vi "TESTER_v1.vi"() -> ()   [LabVIEW 2014, in "PICam.lvlib"]
uses:
  PICam.lvlib
  Ctrls/PicamModel.ctl
  Ctrls/PicamROI.ctl
  Ctrls/ShutterTimingMode.ctl
  Ctrls/PicamAdcQuality.ctl
  Ctrls/PicamADCAnalogGain.ctl
  Ctrls/PicamTriggerResponse.ctl
  Ctrls/PicamTriggerDetermination.ctl
  Ctrls/PicamOutputSignal.ctl
  Ctrls/PicamPixelFormat.ctl
  Ctrls/ReadoutControlMode.ctl
  Ctrls/PicamReadoutOrientation.ctl
  Ctrls/PicamSensorType.ctl
  Ctrls/PicamTimeStamps.ctl
  Ctrls/PicamSensorTemperatureStatus.ctl
  Ctrls/PicamCcdCharacteristics.ctl
  Ctrls/PicamOrientation.ctl
panel:
  in  "PicamTriggerDetemination":T1=2 items=["PositivePolarity"=1, "NegativePolarity"=2, "RisingEdge"=3, "FallingEdge"=4, "AlternatingEdgeRising"=5, "AlternatingEdgeFalling"=6]
  in  "PicamTriggerResponse":T2=1 items=["NoResponse"=1, "ReadoutPerTrigger"=2, "ShiftPerTrigger"=3, "ExposeDuringTriggerPulse"=4, "StartOnSingleTrigger"=5, "GatePerTrigger"=6]
  in  "PicamOutputSignal_":T3=2 items=["NotReadingOut"=1, "ShutterOpen"=2, "Busy"=3, "AlwaysLow"=4, "AlwaysHigh"=5, "Acquiring"=6, "ShiftingUnderMask"=7, "Exposing"=8, "EffectivelyExposing"=9, "ReadingOut"=10, "WaitingForTrigger"=11, "InternalTriggerT0"=12, "Gate"=13, "AuxOutput"=14, "EffectivelyExposingAlternation"=15]
  in  "ReadoutControlMode":T4=1 items=["FullFrame"=1, "FrameTransfer"=2, "Kinetics"=3, "SpectraKinetics"=4, "Interline"=5, "Dif"=6, "SeNsR"=7, "RollingShutter"=8]
  in  "PicamTimeStamps_":T5 items=["None", "ExposureStarted", "ExposureEnded"]
  in  "PicamAdcAnalogGain":T6=2 items=["Low"=1, "Medium"=2, "High"=3]
  in  "PicamAdcQuality":T7=1 items=["LowNoise"=1, "HighCapacity"=2, "ElectronMultiplied"=3, "HighSpeed"=4]
  in  "ShutterTimingMode":T8=1 items=["Normal"=1, "AlwaysClosed"=2, "AlwaysOpen"=3, "OpenBeforeTrigger"=4]
  in  "ReadoutCount":i64=1
  in  "TimeStampResolution":i32=10000000
  in  "CleanUntilTrigger":bool=TRUE
  in  "CleanSerialRegister":bool=TRUE
  in  "TrackFrames":bool
  in  "DisableDataFormatting":bool
  in  "NormalizeOrientation":bool=TRUE
  in  "CleanSectionFinalHeightCount":i32=5
  in  "CleanSectionFinalHeight":i32=2
  in  "CleanCycleHeight":i32=100
  in  "CleanCycleCount":i32=1
  in  "ActiveBottomMargin":i32
  in  "ActiveRightMargin":i32=8
  in  "ActiveTopMargin":i32
  in  "ActiveLeftMargin":i32=8
  in  "ActiveHeight":i32=100
  in  "ActiveWidth":i32=1340
  in  "FrameTrackingBitDepth":i32=64
  in  "TimeStampBitDepth":i32=64
  in  "AdcBitDepth":i32=2
  in  "KineticsWindowHeight":i32=10
  in  "VerticalShiftRate":dbl=15.2
  in  "ShutterClosingDelay":dbl=8.0
  in  "ShutterDelayResolution":dbl=1000.0
  in  "AdcSpeed":dbl=2.0
  in  "SensorTemperatureSetPoint (C)":dbl=-75.0
  in  "ExposureTime (ms)":dbl=300.0
  in  "SET PARAMETERS?":bool
  out "rois":T9[](array[typedef])=[{"x"=1, "width"=1339, "x_binning"=1, "y"=1, "height"=99, "y_binning"=1}]
  out "ExactReadoutCountMaximum":i64=65534
  out "TimeStampResolution":i64=10000000
  out "ReadoutCount":i64=1
  out "TrackFrames":bool
  out "NormalizeOrientation":bool=TRUE
  out "CleanUntilTrigger":bool=TRUE
  out "CleanSerialRegister":bool=TRUE
  out "DisableDataFormatting":bool
  out "Orientation":T10 items=["Normal", "FlippedHorizontally", "FlippedVertically"]
  out "PicamCcdCharacteristics_":T11=3 items=["None", "BackIlluminated", "DeepDepleted", "OpenElectrode", "UVEnhanced", "ExcelonEnabled", "SecondaryMask", "Multiport", "AdvancedInvertedMode", "HighResistivity"]
  out "SensorTemperatureStatus":T12=2 items=["Unlocked"=1, "Locked"=2, "Faulted"=3]
  out "TimeStamps":T5 items=["None", "ExposureStarted", "ExposureEnded"]
  out "Sensor Type":T13=1 items=["CCD"=1, "InGaAs"=2, "CMOS"=3]
  out "ReadoutOrientation_":T14 items=["Normal", "FlippedHorizontally", "FlippedVertically"]
  out "ReadoutControlMode":T4=1 items=["FullFrame"=1, "FrameTransfer"=2, "Kinetics"=3, "SpectraKinetics"=4, "Interline"=5, "Dif"=6, "SeNsR"=7, "RollingShutter"=8]
  out "Pixel Format":T15=1 items=["Monochrome16Bit"=1, "Monochrome32Bit"=2]
  out "SensorTemperatureReading":dbl=-75.0
  out "ReadoutTimeCalculation":dbl=69.37595
  out "ReadoutRateCalculation":dbl=12.923912404306506
  out "PixelWidth":dbl=20.0
  out "PixelHeight":dbl=20.0
  out "PixelGapWidth":dbl
  out "PixelGapHeight":dbl
  out "SensorTemperatureSetPoint":dbl=-75.0
  out "VerticalShiftRate":dbl=15.2
  out "FrameRateCalculation":dbl=12.923912404306506
  out "OnlineReadoutRateCalculation":dbl=12.923912404306506
  out "SensorSecondaryMaskedHeight":i32
  out "SensorSecondaryActiveHeight":i32
  out "SensorMaskedTopMargin":i32
  out "SensorMaskedHeight":i32
  out "SensorMaskedBottomMargin":i32
  out "SensorActiveTopMargin":i32
  out "SensorActiveRightMargin":i32=8
  out "SensorActiveLeftMargin":i32=8
  out "SensorActiveExtendedHeight":i32
  out "SensorActiveBottomMargin":i32
  out "ReadoutStride":i32=265122
  out "PixelBitDepth":i32=16
  out "KineticsWindowHeight":i32=10
  out "FrameTrackingBitDepth":i32=64
  out "FrameStride":i32=265122
  out "FramesPerReadout":i32=1
  out "FrameSize":i32=265122
  out "CleanSectionFinalHeightCount":i32=5
  out "CleanSectionFinalHeight":i32=2
  out "Active Width":i32=1340
  out "ActiveTopMargin":i32
  out "ActiveRightMargin":i32=8
  out "ActiveLeftMargin":i32=8
  out "Active Height":i32=100
  out "CleanCycleCount":i32=1
  out "CleanCycleHeight":i32=100
  out "ActiveBottomMargin":i32
  out "TimestampBitDepth":i32=64
  out "OutputSignal":T3=2 items=["NotReadingOut"=1, "ShutterOpen"=2, "Busy"=3, "AlwaysLow"=4, "AlwaysHigh"=5, "Acquiring"=6, "ShiftingUnderMask"=7, "Exposing"=8, "EffectivelyExposing"=9, "ReadingOut"=10, "WaitingForTrigger"=11, "InternalTriggerT0"=12, "Gate"=13, "AuxOutput"=14, "EffectivelyExposingAlternation"=15]
  out "PicamTriggerDetemination_":T1=2 items=["PositivePolarity"=1, "NegativePolarity"=2, "RisingEdge"=3, "FallingEdge"=4, "AlternatingEdgeRising"=5, "AlternatingEdgeFalling"=6]
  out "PicamTriggerResponse_":T2=1 items=["NoResponse"=1, "ReadoutPerTrigger"=2, "ShiftPerTrigger"=3, "ExposeDuringTriggerPulse"=4, "StartOnSingleTrigger"=5, "GatePerTrigger"=6]
  out "AdcBitDepth":i32
  out "AdcSpeed":dbl=2.0
  out "Sensor Active Width":i32=1340
  out "PicamAdcAnalogGain":T6=2 items=["Low"=1, "Medium"=2, "High"=3]
  out "PicamAdcQuality":T7=1 items=["LowNoise"=1, "HighCapacity"=2, "ElectronMultiplied"=3, "HighSpeed"=4]
  out "Shutter Delay Resolution":dbl=1000.0
  out "Shutter Closing Delay":dbl=8.0
  out "Shutter Timing Mode":T8=1 items=["Normal"=1, "AlwaysClosed"=2, "AlwaysOpen"=3, "OpenBeforeTrigger"=4]
  out "Sensor Active Height":i32=100
  out "Exposure Time":dbl
  out "Raw CCD data":u16[][](graph)
  out "Total pixel number":i32=132561
  in  "PicamROI":T9={"x"=1, "width"=1339, "x_binning"=1, "y"=1, "height"=99, "y_binning"=1}
  out "Frame size (bytes)":i32=265122
  out "PicamModel":T16=5 items=["PicamModel_PIMte1024Series"=1401, "PicamModel_PIMte1024F"=1402, "PicamModel_PIMte1024B"=1403, "PicamModel_PIMte1024BR"=1405, "PicamModel_PIMte1024BUV"=1404, "PicamModel_PIMte1024FTSeries"=1406, "PicamModel_PIMte1024FT"=1407, "PicamModel_PIMte1024BFT"=1408, "PicamModel_PIMte1300Series"=1412, "PicamModel_PIMte1300B"=1413, "PicamModel_PIMte1300R"=1414, "PicamModel_PIMte1300BR"=1415, "PicamModel_PIMte2048Series"=1416, "PicamModel_PIMte2048B"=1417, "PicamModel_PIMte2048BR"=1418, "PicamModel_PIMte2KSeries"=1409, "PicamModel_PIMte2KB"=1410, "PicamModel_PIMte2KBUV"=1411, "PicamModel_PixisSeries"=0, "PicamModel_Pixis100Series"=1, "PicamModel_Pixis100F"=2, "PicamModel_Pixis100B"=6, "PicamModel_Pixis100R"=3, "PicamModel_Pixis100C"=4, "PicamModel_Pixis100BR"=5, "PicamModel_Pixis100BExcelon"=54, "PicamModel_Pixis100BRExcelon"=55, "PicamModel_PixisXO100B"=7, "PicamModel_PixisXO100BR"=8, "PicamModel_PixisXB100B"=68, "PicamModel_PixisXB100BR"=69, "PicamModel_Pixis256Series"=26, "PicamModel_Pixis256F"=27, "PicamModel_Pixis256B"=29, "PicamModel_Pixis256E"=28, "PicamModel_Pixis256BR"=30, "PicamModel_PixisXB256BR"=31, "PicamModel_Pixis400Series"=37, "PicamModel_Pixis400F"=38, "PicamModel_Pixis400B"=40, "PicamModel_Pixis400R"=39, "PicamModel_Pixis400BR"=41, "PicamModel_Pixis400BExcelon"=56, "PicamModel_Pixis400BRExcelon"=57, "PicamModel_PixisXO400B"=42, "PicamModel_PixisXB400BR"=70, "PicamModel_Pixis512Series"=43, "PicamModel_Pixis512F"=44, "PicamModel_Pixis512B"=45, "PicamModel_Pixis512BUV"=46, "PicamModel_Pixis512BExcelon"=58, "PicamModel_PixisXO512F"=49, "PicamModel_PixisXO512B"=50, "PicamModel_PixisXF512F"=48, "PicamModel_PixisXF512B"=47, "PicamModel_Pixis1024Series"=9, "PicamModel_Pixis1024F"=10, "PicamModel_Pixis1024B"=11, "PicamModel_Pixis1024BR"=13, "PicamModel_Pixis1024BUV"=12, "PicamModel_Pixis1024BExcelon"=59, "PicamModel_Pixis1024BRExcelon"=60, "PicamModel_PixisXO1024F"=16, "PicamModel_PixisXO1024B"=14, "PicamModel_PixisXO1024BR"=15, "PicamModel_PixisXF1024F"=17, "PicamModel_PixisXF1024B"=18, "PicamModel_PixisXB1024BR"=71, "PicamModel_Pixis1300Series"=51, "PicamModel_Pixis1300F"=52, "PicamModel_Pixis1300F_2"=75, "PicamModel_Pixis1300B"=53, "PicamModel_Pixis1300BR"=73, "PicamModel_Pixis1300BExcelon"=61, "PicamModel_Pixis1300BRExcelon"=62, "PicamModel_PixisXO1300B"=65, "PicamModel_PixisXF1300B"=66, "PicamModel_PixisXB1300R"=72, "PicamModel_Pixis2048Series"=20, "PicamModel_Pixis2048F"=21, "PicamModel_Pixis2048B"=22, "PicamModel_Pixis2048BR"=67, "PicamModel_Pixis2048BExcelon"=63, "PicamModel_Pixis2048BRExcelon"=74, "PicamModel_PixisXO2048B"=23, "PicamModel_PixisXF2048F"=25, "PicamModel_PixisXF2048B"=24, "PicamModel_Pixis2KSeries"=32, "PicamModel_Pixis2KF"=33, "PicamModel_Pixis2KB"=34, "PicamModel_Pixis2KBUV"=36, "PicamModel_Pixis2KBExcelon"=64, "PicamModel_PixisXO2KB"=35, "PicamModel_QuadroSeries"=100, "PicamModel_Quadro4096"=101, "PicamModel_Quadro4096_2"=103, "PicamModel_Quadro4320"=102, "PicamModel_ProEMSeries"=200, "PicamModel_ProEM512Series"=203, "PicamModel_ProEM512B"=201, "PicamModel_ProEM512BK"=205, "PicamModel_ProEM512BExcelon"=204, "PicamModel_ProEM512BKExcelon"=206, "PicamModel_ProEM1024Series"=207, "PicamModel_ProEM1024B"=202, "PicamModel_ProEM1024BExcelon"=208, "PicamModel_ProEM1600Series"=209, "PicamModel_ProEM1600xx2B"=212, "PicamModel_ProEM1600xx2BExcelon"=210, "PicamModel_ProEM1600xx4B"=213, "PicamModel_ProEM1600xx4BExcelon"=211, "PicamModel_ProEMPlusSeries"=600, "PicamModel_ProEMPlus512Series"=603, "PicamModel_ProEMPlus512B"=601, "PicamModel_ProEMPlus512BK"=605, "PicamModel_ProEMPlus512BExcelon"=604, "PicamModel_ProEMPlus512BKExcelon"=606, "PicamModel_ProEMPlus1024Series"=607, "PicamModel_ProEMPlus1024B"=602, "PicamModel_ProEMPlus1024BExcelon"=608, "PicamModel_ProEMPlus1600Series"=609, "PicamModel_ProEMPlus1600xx2B"=612, "PicamModel_ProEMPlus1600xx2BExcelon"=610, "PicamModel_ProEMPlus1600xx4B"=613, "PicamModel_ProEMPlus1600xx4BExcelon"=611, "PicamModel_ProEMHSSeries"=1200, "PicamModel_ProEMHS512Series"=1201, "PicamModel_ProEMHS512B"=1202, "PicamModel_ProEMHS512BK"=1207, "PicamModel_ProEMHS512BExcelon"=1203, "PicamModel_ProEMHS512BKExcelon"=1208, "PicamModel_ProEMHS1024Series"=1204, "PicamModel_ProEMHS1024B"=1205, "PicamModel_ProEMHS1024BExcelon"=1206, "PicamModel_ProEMHS1024B_2"=1212, "PicamModel_ProEMHS1024BExcelon_2"=1213, "PicamModel_ProEMHS1024B_3"=1214, "PicamModel_ProEMHS1024BExcelon_3"=1215, "PicamModel_ProEMHS1K10Series"=1209, "PicamModel_ProEMHS1KB10"=1210, "PicamModel_ProEMHS1KB10Excelon"=1211, "PicamModel_PIMax3Series"=300, "PicamModel_PIMax31024I"=301, "PicamModel_PIMax31024x256"=302, "PicamModel_PIMax4Series"=700, "PicamModel_PIMax41024ISeries"=703, "PicamModel_PIMax41024I"=701, "PicamModel_PIMax41024IRF"=704, "PicamModel_PIMax41024FSeries"=710, "PicamModel_PIMax41024F"=711, "PicamModel_PIMax41024FRF"=712, "PicamModel_PIMax41024x256Series"=705, "PicamModel_PIMax41024x256"=702, "PicamModel_PIMax41024x256RF"=706, "PicamModel_PIMax42048Series"=716, "PicamModel_PIMax42048F"=717, "PicamModel_PIMax42048B"=718, "PicamModel_PIMax42048FRF"=719, "PicamModel_PIMax42048BRF"=720, "PicamModel_PIMax4512EMSeries"=708, "PicamModel_PIMax4512EM"=707, "PicamModel_PIMax4512BEM"=709, "PicamModel_PIMax41024EMSeries"=713, "PicamModel_PIMax41024EM"=715, "PicamModel_PIMax41024BEM"=714, "PicamModel_PylonSeries"=400, "PicamModel_Pylon100Series"=418, "PicamModel_Pylon100F"=404, "PicamModel_Pylon100B"=401, "PicamModel_Pylon100BR"=407, "PicamModel_Pylon100BExcelon"=425, "PicamModel_Pylon100BRExcelon"=426, "PicamModel_Pylon256Series"=419, "PicamModel_Pylon256F"=409, "PicamModel_Pylon256B"=410, "PicamModel_Pylon256E"=411, "PicamModel_Pylon256BR"=412, "PicamModel_Pylon400Series"=420, "PicamModel_Pylon400F"=405, "PicamModel_Pylon400B"=402, "PicamModel_Pylon400BR"=408, "PicamModel_Pylon400BExcelon"=427, "PicamModel_Pylon400BRExcelon"=428, "PicamModel_Pylon1024Series"=421, "PicamModel_Pylon1024B"=417, "PicamModel_Pylon1024BExcelon"=429, "PicamModel_Pylon1300Series"=422, "PicamModel_Pylon1300F"=406, "PicamModel_Pylon1300B"=403, "PicamModel_Pylon1300R"=438, "PicamModel_Pylon1300BR"=432, "PicamModel_Pylon1300BExcelon"=430, "PicamModel_Pylon1300BRExcelon"=433, "PicamModel_Pylon2048Series"=423, "PicamModel_Pylon2048F"=415, "PicamModel_Pylon2048B"=434, "PicamModel_Pylon2048BR"=416, "PicamModel_Pylon2048BExcelon"=435, "PicamModel_Pylon2048BRExcelon"=436, "PicamModel_Pylon2KSeries"=424, "PicamModel_Pylon2KF"=413, "PicamModel_Pylon2KB"=414, "PicamModel_Pylon2KBUV"=437, "PicamModel_Pylon2KBExcelon"=431, "PicamModel_PylonirSeries"=900, "PicamModel_Pylonir1024Series"=901, "PicamModel_Pylonir102422"=902, "PicamModel_Pylonir102417"=903, "PicamModel_PionirSeries"=500, "PicamModel_Pionir640"=501, "PicamModel_NirvanaSeries"=800, "PicamModel_Nirvana640"=801, "PicamModel_NirvanaSTSeries"=1300, "PicamModel_NirvanaST640"=1301, "PicamModel_NirvanaLNSeries"=1100, "PicamModel_NirvanaLN640"=1101, "PicamModel_SophiaSeries"=1800, "PicamModel_Sophia2048Series"=1801, "PicamModel_Sophia2048B"=1802, "PicamModel_Sophia2048BExcelon"=1803, "PicamModel_SophiaXO2048B"=1804, "PicamModel_SophiaXF2048B"=1805, "PicamModel_SophiaXB2048B"=1806, "PicamModel_Sophia2048135Series"=1807, "PicamModel_Sophia2048135"=1808, "PicamModel_Sophia2048B135"=1809, "PicamModel_Sophia2048BR135"=1810, "PicamModel_Sophia2048B135Excelon"=1811, "PicamModel_Sophia2048BR135Excelon"=1812, "PicamModel_SophiaXO2048B135"=1813, "PicamModel_SophiaXO2048BR135"=1814, "PicamModel_BlazeSeries"=1500, "PicamModel_Blaze100Series"=1507, "PicamModel_Blaze100B"=1501, "PicamModel_Blaze100BR"=1505, "PicamModel_Blaze100HR"=1503, "PicamModel_Blaze100BRLD"=1509, "PicamModel_Blaze100BExcelon"=1511, "PicamModel_Blaze100BRExcelon"=1513, "PicamModel_Blaze100HRExcelon"=1515, "PicamModel_Blaze100BRLDExcelon"=1517, "PicamModel_Blaze400Series"=1508, "PicamModel_Blaze400B"=1502, "PicamModel_Blaze400BR"=1506, "PicamModel_Blaze400HR"=1504, "PicamModel_Blaze400BRLD"=1510, "PicamModel_Blaze400BExcelon"=1512, "PicamModel_Blaze400BRExcelon"=1514, "PicamModel_Blaze400HRExcelon"=1516, "PicamModel_Blaze400BRLDExcelon"=1518, "PicamModel_FergieSeries"=1600, "PicamModel_Fergie256Series"=1601, "PicamModel_Fergie256B"=1602, "PicamModel_Fergie256BR"=1607, "PicamModel_Fergie256BExcelon"=1603, "PicamModel_Fergie256BRExcelon"=1608, "PicamModel_Fergie256FTSeries"=1604, "PicamModel_Fergie256FFT"=1609, "PicamModel_Fergie256BFT"=1605, "PicamModel_Fergie256BRFT"=1610, "PicamModel_Fergie256BFTExcelon"=1606, "PicamModel_Fergie256BRFTExcelon"=1611, "PicamModel_FergieAccessorySeries"=1700, "PicamModel_FergieLampSeries"=1701, "PicamModel_FergieAEL"=1702, "PicamModel_FergieQTH"=1703, "PicamModel_FergieLaserSeries"=1704, "PicamModel_FergieLaser785"=1705, "PicamModel_KuroSeries"=1900, "PicamModel_Kuro1200B"=1901, "PicamModel_Kuro1608B"=1902, "PicamModel_Kuro2048B"=1903]
  out "Camera detected?":bool=TRUE
  out "Serial":string="0205070001"
  out "Sensor name":string="E2V 1340 x 100 (CCD 36)(B)(R)"
  in  "cam index":i32
  out "PICam version":string="5.7.1.1903"
  out "error out":errorcluster
  # "GET INFORMATION / PARAMETER VALUES:"
  # "PIXIS SDK"
  # "Can be set greater than 1340?"
  # "Can be set greater than 100?"
  # "Less important?\n\n- Picam_DestroyString()\n- Picam_GetEnumnerationString()\n- Picam_DestroyCameraIDs()\n- Picam_GetUnavailableCameraIDs()\n+ other Destroy-methods and gettype methods"
  # "To implement:\n\n- Picam_IsLibraryInitialized()\n- Picam_IsCameraIDConnected()\n- Picam_IsCameraIDOpenElsewhere()\n- Picam_DestroyHandles()\n- Picam_GetOpenCameras()\n- Picam_IsCameraConnected()\n- Picam_IsCameraFaulted()\n- Picam_GetFirmwareDetails()\n- Picam_CanSetParameterOnline()\n- Picam_CanReadParameter() \n- Picam_CanWaitForStatusParameter()\n- Picam_GetStatusParameterPurview()\n- Picam_EstimateTimeToStatusParameterValue()\n- Picam_WaitForStatusParameterValue()\n- Picam_CommitParameters()\n- Picam_AreParametersCommited()\n- Picam_WaitForAcquisitionUpdate()\n- PicamAdvanced_GetAcquisitionBuffer()\n- PicamAdvanced_SetAcquisitionBuffer()\n- PicamAdvanced_HasAcquisitionBufferOverrun()"
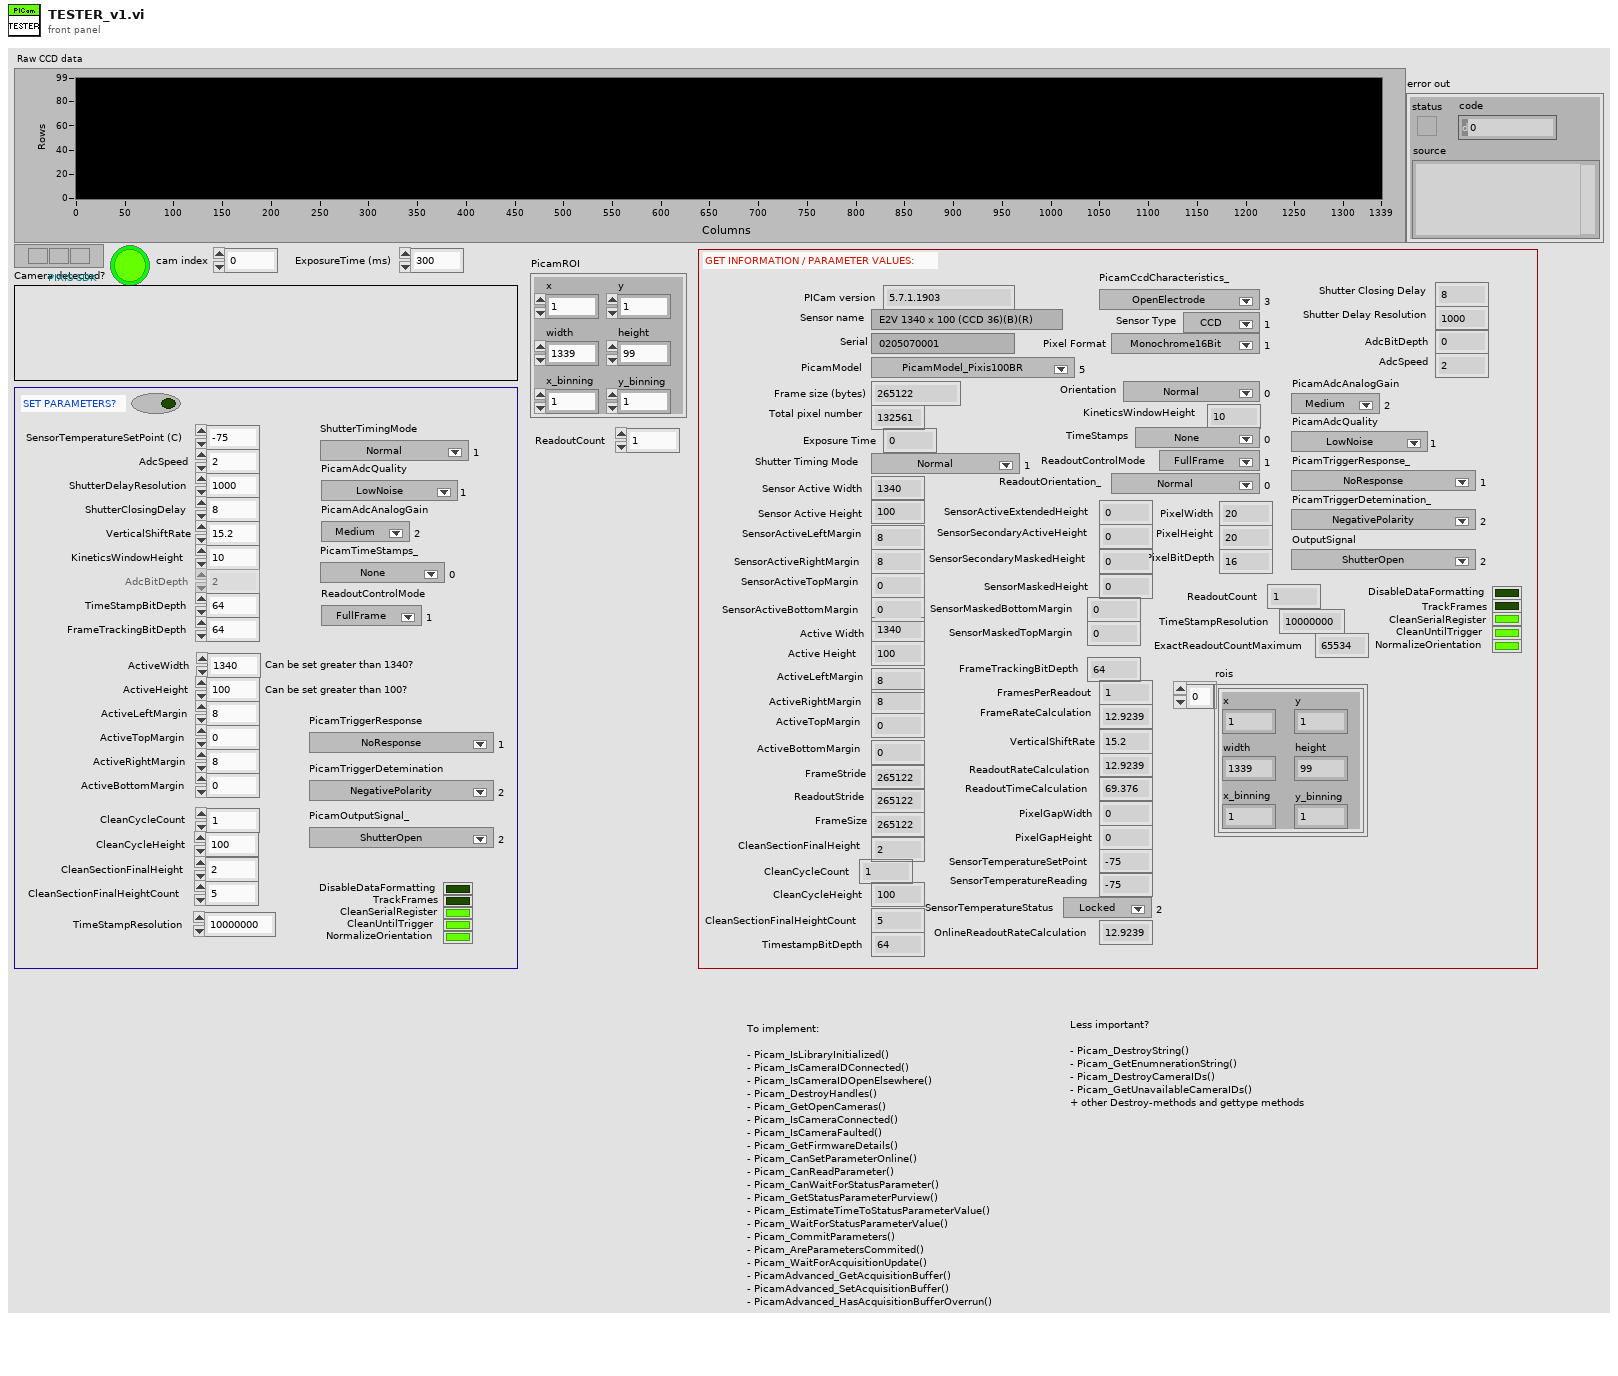
[diagram p1: front panel]
types:
  T1 = typedef "PICam.lvlib/PicamTriggerDetermination.ctl" = u32
  T2 = typedef "PICam.lvlib/PicamTriggerResponse.ctl" = u32
  T3 = typedef "PICam.lvlib/PicamOutputSignal.ctl" = u32
  T4 = typedef "PICam.lvlib/ReadoutControlMode.ctl" = u32
  T5 = typedef "PICam.lvlib/PicamTimeStamps.ctl" = u32
  T6 = typedef "PICam.lvlib/PicamADCAnalogGain.ctl" = u32
  T7 = typedef "PICam.lvlib/PicamAdcQuality.ctl" = u32
  T8 = typedef "PICam.lvlib/ShutterTimingMode.ctl" = u32
  T9 = typedef "PICam.lvlib/PicamROI.ctl" = cluster{"x":i32, "width":i32, "x_binning":i32, "y":i32, "height":i32, "y_binning":i32}
  T10 = typedef "PICam.lvlib/PicamOrientation.ctl" = u32
  T11 = typedef "PICam.lvlib/PicamCcdCharacteristics.ctl" = u32
  T12 = typedef "PICam.lvlib/PicamSensorTemperatureStatus.ctl" = u32
  T13 = typedef "PICam.lvlib/PicamSensorType.ctl" = u32
  T14 = typedef "PICam.lvlib/PicamReadoutOrientation.ctl" = u32
  T15 = typedef "PICam.lvlib/PicamPixelFormat.ctl" = u32
  T16 = typedef "PICAM.lvlib/PicamModel.ctl" = u32
  T17 = typedef "PICam.lvlib/PicamCameraID.ctl" = cluster{"PicamModel":T16, "PicamComputerInterface":T18, "sensor_name":T19, "serial_number":T20}
  T18 = typedef "PICAM.lvlib/PicamComputerInterface.ctl" = u32
  T19 = typedef "PICAM.lvlib/sensor_name.ctl" = cluster{"U8":u8, "U8 2":u8, "U8 3":u8, "U8 4":u8, "U8 5":u8, "U8 6":u8, "U8 7":u8, "U8 8":u8, "U8 9":u8, "U8 10":u8, "U8 11":u8, "U8 12":u8, "U8 13":u8, "U8 14":u8, "U8 15":u8, "U8 16":u8, "U8 17":u8, "U8 18":u8, "U8 19":u8, "U8 20":u8, "U8 21":u8, "U8 22":u8, "U8 23":u8, "U8 24":u8, "U8 25":u8, "U8 26":u8, "U8 27":u8, "U8 28":u8, "U8 29":u8, "U8 30":u8, "U8 31":u8, "U8 32":u8, "U8 33":u8, "U8 34":u8, "U8 35":u8, "U8 36":u8, "U8 37":u8, "U8 38":u8, "U8 39":u8, "U8 40":u8, "U8 41":u8, "U8 42":u8, "U8 43":u8, "U8 44":u8, "U8 45":u8, "U8 46":u8, "U8 47":u8, "U8 48":u8, "U8 49":u8, "U8 50":u8, "U8 51":u8, "U8 52":u8, "U8 53":u8, "U8 54":u8, "U8 55":u8, "U8 56":u8, "U8 57":u8, "U8 58":u8, "U8 59":u8, "U8 60":u8, "U8 61":u8, "U8 62":u8, "U8 63":u8, "U8 64":u8}
  T20 = typedef "PICAM.lvlib/serial_number.ctl" = cluster{"U8":u8, "U8 2":u8, "U8 3":u8, "U8 4":u8, "U8 5":u8, "U8 6":u8, "U8 7":u8, "U8 8":u8, "U8 9":u8, "U8 10":u8, "U8 11":u8, "U8 12":u8, "U8 13":u8, "U8 14":u8, "U8 15":u8, "U8 16":u8, "U8 17":u8, "U8 18":u8, "U8 19":u8, "U8 20":u8, "U8 21":u8, "U8 22":u8, "U8 23":u8, "U8 24":u8, "U8 25":u8, "U8 26":u8, "U8 27":u8, "U8 28":u8, "U8 29":u8, "U8 30":u8, "U8 31":u8, "U8 32":u8, "U8 33":u8, "U8 34":u8, "U8 35":u8, "U8 36":u8, "U8 37":u8, "U8 38":u8, "U8 39":u8, "U8 40":u8, "U8 41":u8, "U8 42":u8, "U8 43":u8, "U8 44":u8, "U8 45":u8, "U8 46":u8, "U8 47":u8, "U8 48":u8, "U8 49":u8, "U8 50":u8, "U8 51":u8, "U8 52":u8, "U8 53":u8, "U8 54":u8, "U8 55":u8, "U8 56":u8, "U8 57":u8, "U8 58":u8, "U8 59":u8, "U8 60":u8, "U8 61":u8, "U8 62":u8, "U8 63":u8, "U8 64":u8}
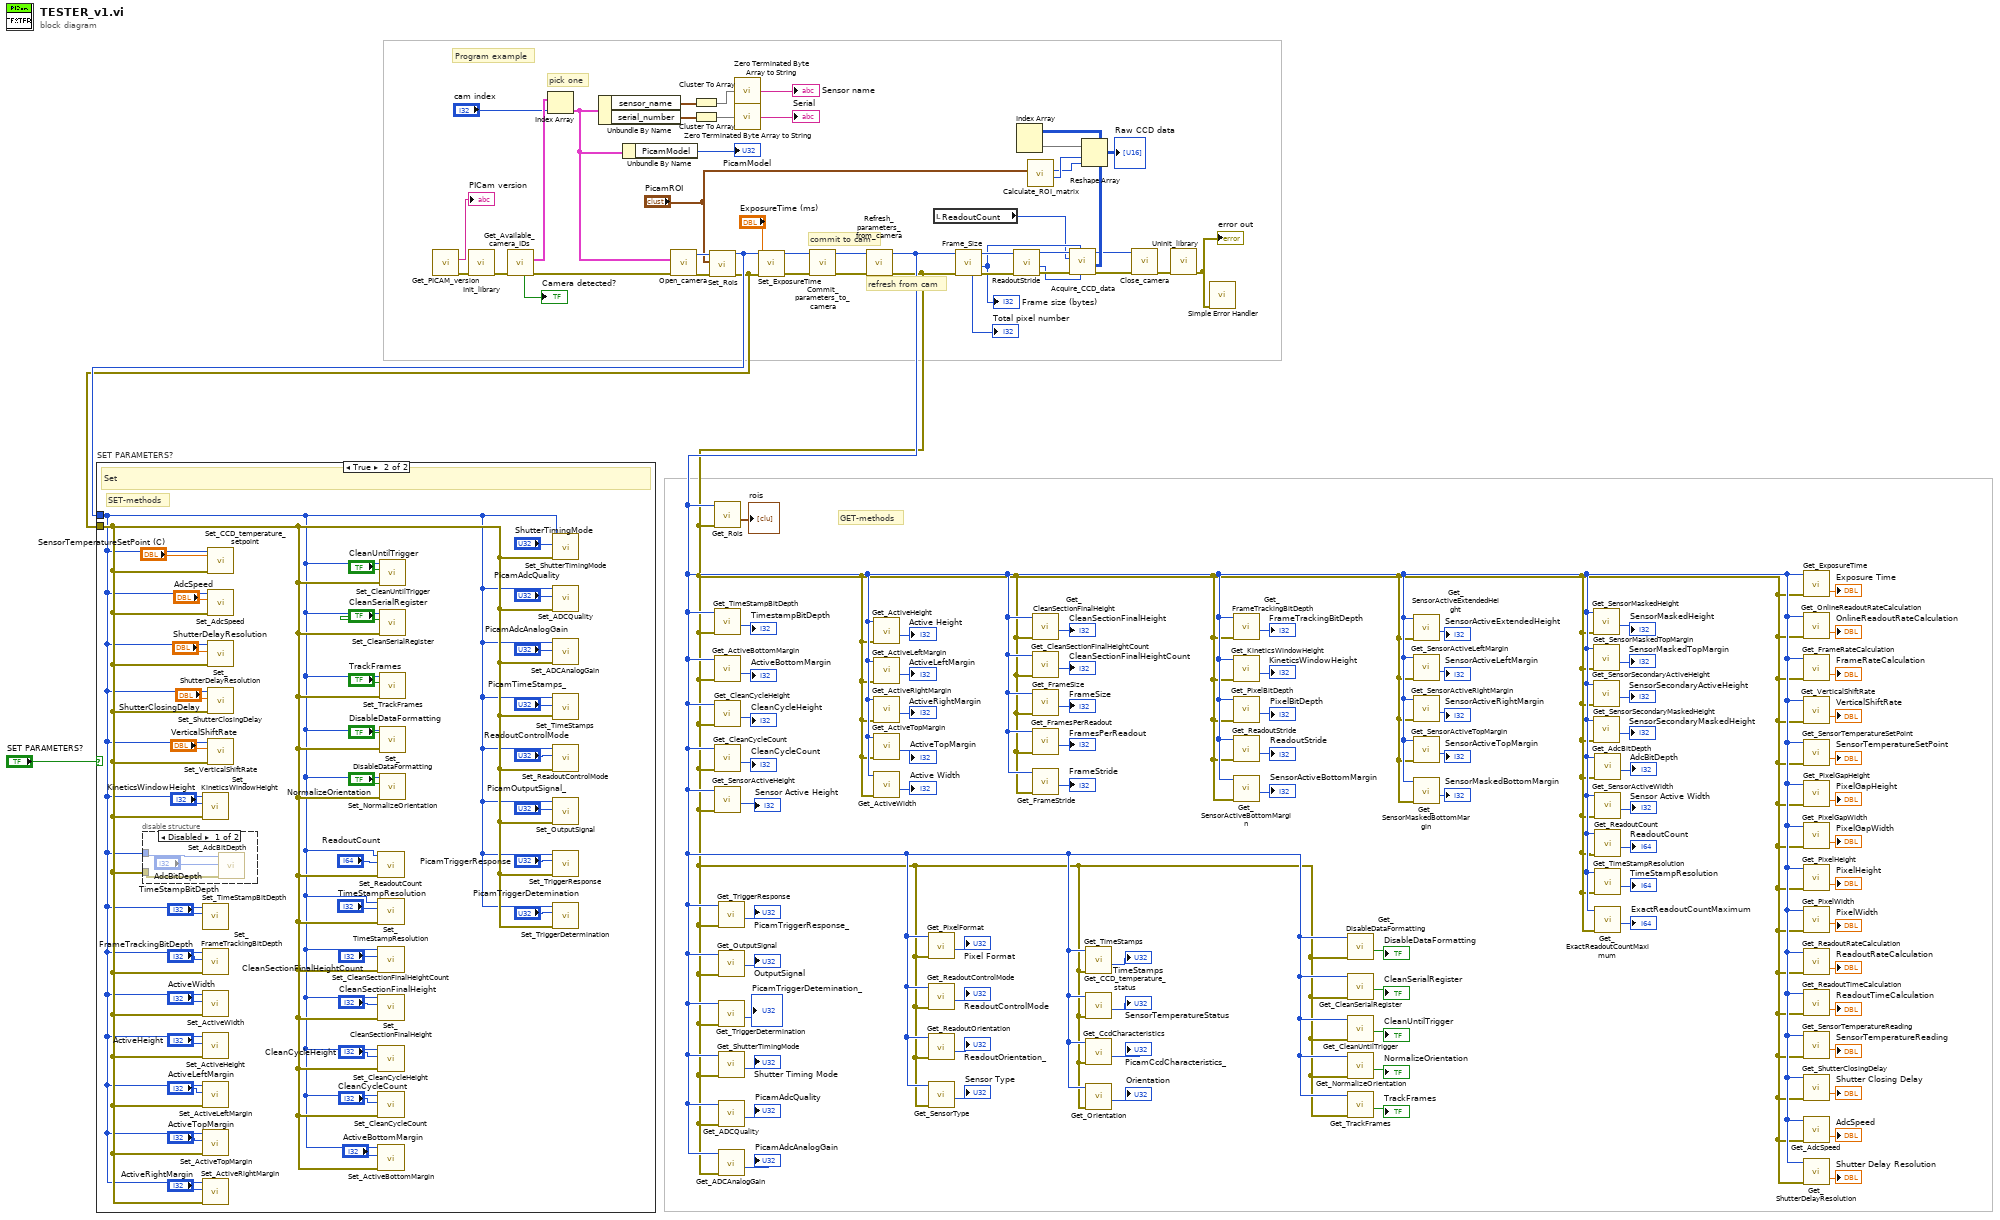
[diagram p0: block diagram]
diagram:
  # "GET-methods"
  # "Program example"
  # "refresh from cam"
  # "commit to cam"
  # "pick one"
  n1 = call "Get_PICAM_version.vi"() -> ("error out"=w114:errorcluster, "PICam version"=→"PICam version":string)  [unwired: 10 in]
  n2 = call "Init_library.vi"("error in"=w114) -> ("error out"=w112:errorcluster)  [unwired: 10 in]
  n3 = call "Get_Available_camera_IDs.vi"("error in"=w112) -> ("error out"=w100:errorcluster, "PicamCameraIDs"=w111:T17[], "Camera detected?"=→"Camera detected?":bool)  [unwired: 8 in]
  n4 = Index Array(array=w111, index="cam index") -> (element=w101:T17)
  n5 = Unbundle By Name(w101) -> ("sensor_name"=w109:T19, "serial_number"=w108:T20)
  n6 = Unbundle By Name(w101) -> ("PicamModel"=→"PicamModel":T16)
  n7 = call "Open_camera.vi"("error in"=w100, "PicamCameraID"=w101) -> ("error out"=w7:errorcluster, "camera handler out"=w86:u64)  [unwired: 8 in]
  n8 = Cluster To Array(cluster=w109) -> (array=w107:u8[])
  n9 = Cluster To Array(cluster=w108) -> (array=w106:u8[])
  n10 = call "Set_Rois.vi"("error in"=w7, "PicamROI"="PicamROI", "camera handle in"=w86) -> ("error out"=w2:errorcluster, "camera handle out"=w3:u64)  [unwired: 7 in]
  n11 = case "SET PARAMETERS?" shown="True" "SET PARAMETERS?" {
    tunnel: w3 -> [_ w115]
    tunnel: w2 -> [_ w116]
    frame False {
      # "Don't set"
    }
    frame True {
      # "SET-methods"
      # "Set"
      n12 = disable-structure shown="Disabled" {
        disable-tunnel: w115 -> [w151 _]
        disable-tunnel: w116 -> [w150 _]
        frame Disabled {
          n13 = call "Set_AdcBitDepth.vi"("error in"=w150, "AdcBitDepth"="AdcBitDepth", "camera handle in"=w151) -> ()  [unwired: 7 in, 2 out]
        }
        frame Enabled {
        }
      }
      n14 = call "Set_KineticsWindowHeight.vi"("error in"=w116, "KineticsWindowHeight"="KineticsWindowHeight", "camera handle in"=w115) -> ()  [unwired: 7 in, 2 out]
      n15 = call "Set_TimeStampBitDepth.vi"("TimeStampBitDepth"="TimeStampBitDepth", "camera handle in"=w115) -> ()  [unwired: 8 in, 2 out]
      n16 = call "Set_FrameTrackingBitDepth.vi"("error in"=w116, "FrameTrackingBitDepth"="FrameTrackingBitDepth", "camera handle in"=w115) -> ()  [unwired: 7 in, 2 out]
      n17 = call "Set_ActiveWidth.vi"("error in"=w116, "ActiveWidth"="ActiveWidth", "camera handle in"=w115) -> ()  [unwired: 7 in, 2 out]
      n18 = call "Set_ActiveHeight.vi"("error in"=w116, "ActiveHeight"="ActiveHeight", "camera handle in"=w115) -> ()  [unwired: 7 in, 2 out]
      n19 = call "Set_ActiveLeftMargin.vi"("error in"=w116, "ActiveLeftMargin"="ActiveLeftMargin", "camera handle in"=w115) -> ()  [unwired: 7 in, 2 out]
      n20 = call "Set_ActiveTopMargin.vi"("error in"=w116, "ActiveTopMargin"="ActiveTopMargin", "camera handle in"=w115) -> ()  [unwired: 7 in, 2 out]
      n21 = call "Set_ActiveRightMargin.vi"("error in"=w116, "ActiveRightMargin"="ActiveRightMargin", "camera handle in"=w115) -> ()  [unwired: 7 in, 2 out]
      n22 = call "Set_CCD_temperature_setpoint.vi"("error in"=w116, "SensorTemperatureSetPoint (C)"="SensorTemperatureSetPoint (C)", "camera handle in"=w115) -> ()  [unwired: 7 in, 2 out]
      n23 = call "Set_AdcSpeed.vi"("error in"=w116, "AdcSpeed"="AdcSpeed", "camera handle in"=w115) -> ()  [unwired: 7 in, 2 out]
      n24 = call "Set_ShutterDelayResolution.vi"("error in"=w116, "ShutterDelayResolution"="ShutterDelayResolution", "camera handle in"=w115) -> ()  [unwired: 7 in, 2 out]
      n25 = call "Set_ShutterClosingDelay.vi"("error in"=w116, "ShutterClosingDelay"="ShutterClosingDelay", "camera handle in"=w115) -> ()  [unwired: 7 in, 2 out]
      n26 = call "Set_VerticalShiftRate.vi"("error in"=w116, "VerticalShiftRate"="VerticalShiftRate", "camera handle in"=w115) -> ()  [unwired: 7 in, 2 out]
      n27 = call "Set_ReadoutCount.vi"("error in"=w116, "ReadoutCount"="ReadoutCount", "camera handle in"=w115) -> ()  [unwired: 7 in, 2 out]
      n28 = call "Set_TimeStampResolution.vi"("error in"=w116, "TimeStampResolution"="TimeStampResolution", "camera handle in"=w115) -> ()  [unwired: 7 in, 2 out]
      n29 = call "Set_CleanSectionFinalHeightCount.vi"("error in"=w116, "CleanSectionFinalHeightCount"="CleanSectionFinalHeightCount", "camera handle in"=w115) -> ()  [unwired: 7 in, 2 out]
      n30 = call "Set_CleanSectionFinalHeight.vi"("error in"=w116, "CleanSectionFinalHeight"="CleanSectionFinalHeight", "camera handle in"=w115) -> ()  [unwired: 7 in, 2 out]
      n31 = call "Set_CleanCycleHeight.vi"("error in"=w116, "CleanCycleHeight"="CleanCycleHeight", "camera handle in"=w115) -> ()  [unwired: 7 in, 2 out]
      n32 = call "Set_CleanCycleCount.vi"("error in"=w116, "CleanCycleCount"="CleanCycleCount", "camera handle in"=w115) -> ()  [unwired: 7 in, 2 out]
      n33 = call "Set_ActiveBottomMargin.vi"("error in"=w116, "ActiveBottomMargin"="ActiveBottomMargin", "camera handle in"=w115) -> ()  [unwired: 7 in, 2 out]
      n34 = call "Set_CleanUntilTrigger.vi"("error in"=w116, "CleanUntilTrigger"="CleanUntilTrigger", "camera handle in"=w115) -> ()  [unwired: 7 in, 2 out]
      n35 = call "Set_CleanSerialRegister.vi"("error in"=w116, "CleanSerialRegister"="CleanSerialRegister", "camera handle in"=w115) -> ()  [unwired: 7 in, 2 out]
      n36 = call "Set_TrackFrames.vi"("error in"=w116, "TrackFrames"="TrackFrames", "camera handle in"=w115) -> ()  [unwired: 7 in, 2 out]
      n37 = call "Set_DisableDataFormatting.vi"("error in"=w116, "DisableDataFormatting"="DisableDataFormatting", "camera handle in"=w115) -> ()  [unwired: 7 in, 2 out]
      n38 = call "Set_NormalizeOrientation.vi"("error in"=w116, "NormalizeOrientation"="NormalizeOrientation", "camera handle in"=w115) -> ()  [unwired: 7 in, 2 out]
      n39 = call "Set_ShutterTimingMode.vi"("error in"=w116, "ShutterTimingMode"="ShutterTimingMode", "camera handle in"=w115) -> ()  [unwired: 7 in, 2 out]
      n40 = call "Set_ADCQuality.vi"("error in"=w116, "PicamAdcQuality"="PicamAdcQuality", "camera handle in"=w115) -> ()  [unwired: 7 in, 2 out]
      n41 = call "Set_ADCAnalogGain.vi"("error in"=w116, "PicamAdcAnalogGain"="PicamAdcAnalogGain", "camera handle in"=w115) -> ()  [unwired: 7 in, 2 out]
      n42 = call "Set_TimeStamps.vi"("error in"=w116, "PicamTimeStamps_"="PicamTimeStamps_", "camera handle in"=w115) -> ()  [unwired: 7 in, 2 out]
      n43 = call "Set_ReadoutControlMode.vi"("error in"=w116, "ReadoutControlMode"="ReadoutControlMode", "camera handle in"=w115) -> ()  [unwired: 7 in, 2 out]
      n44 = call "Set_OutputSignal.vi"("error in"=w116, "PicamOutputSignal_"="PicamOutputSignal_", "camera handle in"=w115) -> ()  [unwired: 7 in, 2 out]
      n45 = call "Set_TriggerResponse.vi"("error in"=w116, "PicamTriggerResponse_"="PicamTriggerResponse", "camera handle in"=w115) -> ()  [unwired: 7 in, 2 out]
      n46 = call "Set_TriggerDetermination.vi"("error in"=w116, "PicamTriggerDetemination_"="PicamTriggerDetemination", "camera handle in"=w115) -> ()  [unwired: 7 in, 2 out]
    }
  }
  n47 = call "Zero Terminated Byte Array to String.vi"("byte array"=w107) -> ("string"=→"Sensor name":string)  [unwired: 4 in]
  n48 = call "Zero Terminated Byte Array to String.vi"("byte array"=w106) -> ("string"=→"Serial":string)  [unwired: 4 in]
  n49 = call "Set_ExposureTime.vi"("error in"=w2, "ExposureTime (ms)"="ExposureTime (ms)", "camera handle in"=w3) -> ("error out"=w5:errorcluster, "camera handle out"=w33:u64)  [unwired: 7 in]
  n50 = call "Commit_parameters_to_camera.vi"("error in"=w5, "camera handle in"=w33) -> ("error out"=w87:errorcluster, "camera handle out"=w88:u64)  [unwired: 8 in]
  n51 = call "Refresh_parameters_from_camera.vi"("error in"=w87, "camera handle in"=w88) -> ("error out"=w1:errorcluster, "camera handle out"=w4:u64)  [unwired: 8 in]
  n52 = call "Get_Rois.vi"("error in"=w1, "camera handle in"=w4) -> ("rois"=→"rois":T9[])  [unwired: 7 in, 2 out]
  n53 = call "Get_TimeStampBitDepth.vi"("error in"=w1, "camera handle in"=w4) -> ("TimestampBitDepth"=→"TimestampBitDepth":i32)  [unwired: 7 in, 2 out]
  n54 = call "Get_ActiveBottomMargin.vi"("error in"=w1, "camera handle in"=w4) -> ("ActiveBottomMargin"=→"ActiveBottomMargin":i32)  [unwired: 7 in, 2 out]
  n55 = call "Get_CleanCycleHeight.vi"("error in"=w1, "camera handle in"=w4) -> ("CleanCycleHeight"=→"CleanCycleHeight":i32)  [unwired: 7 in, 2 out]
  n56 = call "Get_CleanCycleCount.vi"("error in"=w1, "camera handle in"=w4) -> ("CleanCycleCount"=→"CleanCycleCount":i32)  [unwired: 7 in, 2 out]
  n57 = call "Get_SensorActiveHeight.vi"("error in"=w1, "camera handle in"=w4) -> ("SensorActiveHeight"=→"Sensor Active Height":i32)  [unwired: 7 in, 2 out]
  n58 = call "Get_TriggerResponse.vi"("error in"=w1, "camera handle in"=w4) -> ("PicamTriggerResponse_"=→"PicamTriggerResponse_":T2)  [unwired: 7 in, 2 out]
  n59 = call "Get_OutputSignal.vi"("error in"=w1, "camera handle in"=w4) -> ("PicamOutputSignal_"=→"OutputSignal":T3)  [unwired: 7 in, 2 out]
  n60 = call "Get_TriggerDetermination.vi"("error in"=w1, "camera handle in"=w4) -> ("PicamTriggerDetemination_"=→"PicamTriggerDetemination_":T1)  [unwired: 7 in, 2 out]
  n61 = call "Get_ShutterTimingMode.vi"("error in"=w1, "camera handle in"=w4) -> ("ShutterTimingMode"=→"Shutter Timing Mode":T8)  [unwired: 7 in, 2 out]
  n62 = call "Get_ADCQuality.vi"("error in"=w1, "camera handle in"=w4) -> ("PicamAdcQuality"=→"PicamAdcQuality":T7)  [unwired: 7 in, 2 out]
  n63 = call "Get_ADCAnalogGain.vi"("error in"=w1, "camera handle in"=w4) -> ("PicamAdcAnalogGain"=→"PicamAdcAnalogGain":T6)  [unwired: 7 in, 2 out]
  n64 = call "Get_ActiveHeight.vi"("error in"=w1, "camera handle in"=w4) -> ("ActiveHeight"=→"Active Height":i32)  [unwired: 7 in, 2 out]
  n65 = call "Get_ActiveLeftMargin.vi"("error in"=w1, "camera handle in"=w4) -> ("ActiveLeftMargin"=→"ActiveLeftMargin":i32)  [unwired: 7 in, 2 out]
  n66 = call "Get_ActiveRightMargin.vi"("error in"=w1, "camera handle in"=w4) -> ("ActiveRightMargin"=→"ActiveRightMargin":i32)  [unwired: 7 in, 2 out]
  n67 = call "Get_ActiveTopMargin.vi"("error in"=w1, "camera handle in"=w4) -> ("ActiveTopMargin"=→"ActiveTopMargin":i32)  [unwired: 7 in, 2 out]
  n68 = call "Get_ActiveWidth.vi"("error in"=w1, "camera handle in"=w4) -> ("ActiveWidth"=→"Active Width":i32)  [unwired: 7 in, 2 out]
  n69 = call "Get_PixelFormat.vi"("error in"=w1, "camera handle in"=w4) -> ("PicamPixelFormat_"=→"Pixel Format":T15)  [unwired: 7 in, 2 out]
  n70 = call "Get_ReadoutControlMode.vi"("error in"=w1, "camera handle in"=w4) -> ("ReadoutControlMode"=→"ReadoutControlMode":T4)  [unwired: 7 in, 2 out]
  n71 = call "Get_ReadoutOrientation.vi"("error in"=w1, "camera handle in"=w4) -> ("PicamReadoutOrientation_"=→"ReadoutOrientation_":T14)  [unwired: 7 in, 2 out]
  n72 = call "Get_SensorType.vi"("error in"=w1, "camera handle in"=w4) -> ("PicamSensorType_"=→"Sensor Type":T13)  [unwired: 7 in, 2 out]
  n73 = local read "ReadoutCount"() -> (w22:i64)
  n74 = call "Frame_Size.vi"("error in"=w1, "camera handle in"=w4) -> ("error out"=w96:errorcluster, "Frame size (bytes)"=w25:i32, "camera handle out"=w97:u64, "Total pixel number"=→"Total pixel number":i32)  [unwired: 5 in, 1 out]
  "Frame size (bytes)" <- w25
  n75 = call "ReadoutStride.vi"("error in"=w96, "camera handle in"=w97) -> ("error out"=w94:errorcluster, "ReadoutStride (bytes)"=w24:i32, "camera handle out"=w95:u64)  [unwired: 7 in]
  n76 = call "Calculate_ROI_matrix.vi"("PicamROI"="PicamROI") -> ("Columns (pixels)"=w90:i32, "Rows (pixels)"=w89:i32)  [unwired: 8 in, 1 out]
  n77 = call "Get_CleanSectionFinalHeight.vi"("error in"=w1, "camera handle in"=w4) -> ("CleanSectionFinalHeight"=→"CleanSectionFinalHeight":i32)  [unwired: 7 in, 2 out]
  n78 = call "Get_CleanSectionFinalHeightCount.vi"("error in"=w1, "camera handle in"=w4) -> ("CleanSectionFinalHeightCount"=→"CleanSectionFinalHeightCount":i32)  [unwired: 7 in, 2 out]
  n79 = call "Get_FrameSize.vi"("error in"=w1, "camera handle in"=w4) -> ("FrameSize"=→"FrameSize":i32)  [unwired: 7 in, 2 out]
  n80 = call "Get_FramesPerReadout.vi"("error in"=w1, "camera handle in"=w4) -> ("FramesPerReadout"=→"FramesPerReadout":i32)  [unwired: 7 in, 2 out]
  n81 = call "Get_FrameStride.vi"("error in"=w1, "camera handle in"=w4) -> ("FrameStride"=→"FrameStride":i32)  [unwired: 7 in, 2 out]
  n82 = call "Acquire_CCD_data.vi"("readout_stride (bytes)"=w24, "frame size (bytes)"=w25, "error in"=w94, "readout_count"=w22, "camera handle in"=w95) -> ("error out"=w23:errorcluster, "read_count * frames"=w92:u16[][], "camera handle out"=w6:u64)  [unwired: 3 in, 1 out]
  n83 = Index Array(array=w92) -> (element=w93:u16[])  [unwired: 2 in]
  n84 = Reshape Array(w93, w90, w89) -> (→"Raw CCD data":u16[][])
  n85 = call "Get_TimeStamps.vi"("error in"=w1, "camera handle in"=w4) -> ("PicamTimeStamps_"=→"TimeStamps":T5)  [unwired: 7 in, 2 out]
  n86 = call "Get_CCD_temperature_status.vi"("error in"=w1, "camera handle in"=w4) -> ("PicamSensorTemperatureStatus"=→"SensorTemperatureStatus":T12)  [unwired: 7 in, 2 out]
  n87 = call "Get_CcdCharacteristics.vi"("error in"=w1, "camera handle in"=w4) -> ("PicamCcdCharacteristics_"=→"PicamCcdCharacteristics_":T11)  [unwired: 7 in, 2 out]
  n88 = call "Get_Orientation.vi"("error in"=w1, "camera handle in"=w4) -> ("PicamOrientation_"=→"Orientation":T10)  [unwired: 7 in, 2 out]
  n89 = call "Close_camera.vi"("error in"=w23, "camera handle in"=w6) -> ("error out"=w99:errorcluster)  [unwired: 9 in]
  n90 = call "Uninit_library.vi"("error in"=w99) -> ("error out"=w27:errorcluster)  [unwired: 10 in]
  "error out" <- w27
  n91 = call <vilib>:"Simple Error Handler.vi"("error in (no error)"=w27) -> ()  [unwired: 4 in, 5 out]
  n92 = call "Get_FrameTrackingBitDepth.vi"("error in"=w1, "camera handle in"=w4) -> ("FrameTrackingBitDepth"=→"FrameTrackingBitDepth":i32)  [unwired: 7 in, 2 out]
  n93 = call "Get_KineticsWindowHeight.vi"("error in"=w1, "camera handle in"=w4) -> ("KineticsWindowHeight"=→"KineticsWindowHeight":i32)  [unwired: 7 in, 2 out]
  n94 = call "Get_PixelBitDepth.vi"("error in"=w1, "camera handle in"=w4) -> ("PixelBitDepth"=→"PixelBitDepth":i32)  [unwired: 7 in, 2 out]
  n95 = call "Get_ReadoutStride.vi"("error in"=w1, "camera handle in"=w4) -> ("ReadoutStride"=→"ReadoutStride":i32)  [unwired: 7 in, 2 out]
  n96 = call "Get_SensorActiveBottomMargin.vi"("error in"=w1, "camera handle in"=w4) -> ("SensorActiveBottomMargin"=→"SensorActiveBottomMargin":i32)  [unwired: 7 in, 2 out]
  n97 = call "Get_DisableDataFormatting.vi"("error in"=w1, "camera handle in"=w4) -> ("DisableDataFormatting"=→"DisableDataFormatting":bool)  [unwired: 7 in, 2 out]
  n98 = call "Get_CleanSerialRegister.vi"("error in"=w1, "camera handle in"=w4) -> ("CleanSerialRegister"=→"CleanSerialRegister":bool)  [unwired: 7 in, 2 out]
  n99 = call "Get_CleanUntilTrigger.vi"("error in"=w1, "camera handle in"=w4) -> ("CleanUntilTrigger"=→"CleanUntilTrigger":bool)  [unwired: 7 in, 2 out]
  n100 = call "Get_NormalizeOrientation.vi"("error in"=w1, "camera handle in"=w4) -> ("NormalizeOrientation"=→"NormalizeOrientation":bool)  [unwired: 7 in, 2 out]
  n101 = call "Get_TrackFrames.vi"("error in"=w1, "camera handle in"=w4) -> ("TrackFrames"=→"TrackFrames":bool)  [unwired: 7 in, 2 out]
  n102 = call "Get_SensorActiveExtendedHeight.vi"("error in"=w1, "camera handle in"=w4) -> ("SensorActiveExtendedHeight"=→"SensorActiveExtendedHeight":i32)  [unwired: 7 in, 2 out]
  n103 = call "Get_SensorActiveLeftMargin.vi"("error in"=w1, "camera handle in"=w4) -> ("SensorActiveLeftMargin"=→"SensorActiveLeftMargin":i32)  [unwired: 7 in, 2 out]
  n104 = call "Get_SensorActiveRightMargin.vi"("error in"=w1, "camera handle in"=w4) -> ("SensorActiveRightMargin"=→"SensorActiveRightMargin":i32)  [unwired: 7 in, 2 out]
  n105 = call "Get_SensorActiveTopMargin.vi"("error in"=w1, "camera handle in"=w4) -> ("SensorActiveTopMargin"=→"SensorActiveTopMargin":i32)  [unwired: 7 in, 2 out]
  n106 = call "Get_SensorMaskedBottomMargin.vi"("error in"=w1, "camera handle in"=w4) -> ("SensorMaskedBottomMargin"=→"SensorMaskedBottomMargin":i32)  [unwired: 7 in, 2 out]
  n107 = call "Get_SensorMaskedHeight.vi"("error in"=w1, "camera handle in"=w4) -> ("SensorMaskedHeight"=→"SensorMaskedHeight":i32)  [unwired: 7 in, 2 out]
  n108 = call "Get_SensorMaskedTopMargin.vi"("error in"=w1, "camera handle in"=w4) -> ("SensorMaskedTopMargin"=→"SensorMaskedTopMargin":i32)  [unwired: 7 in, 2 out]
  n109 = call "Get_SensorSecondaryActiveHeight.vi"("error in"=w1, "camera handle in"=w4) -> ("SensorSecondaryActiveHeight"=→"SensorSecondaryActiveHeight":i32)  [unwired: 7 in, 2 out]
  n110 = call "Get_SensorSecondaryMaskedHeight.vi"("error in"=w1, "camera handle in"=w4) -> ("SensorSecondaryMaskedHeight"=→"SensorSecondaryMaskedHeight":i32)  [unwired: 7 in, 2 out]
  n111 = call "Get_AdcBitDepth.vi"("error in"=w1, "camera handle in"=w4) -> ("AdcBitDepth"=→"AdcBitDepth":i32)  [unwired: 7 in, 2 out]
  n112 = call "Get_SensorActiveWidth.vi"("error in"=w1, "camera handle in"=w4) -> ("Sensor Active Width"=→"Sensor Active Width":i32)  [unwired: 7 in, 2 out]
  n113 = call "Get_ReadoutCount.vi"("error in"=w1, "camera handle in"=w4) -> ("ReadoutCount"=→"ReadoutCount":i64)  [unwired: 7 in, 2 out]
  n114 = call "Get_TimeStampResolution.vi"("error in"=w1, "camera handle in"=w4) -> ("TimeStampResolution"=→"TimeStampResolution":i64)  [unwired: 7 in, 2 out]
  n115 = call "Get_ExactReadoutCountMaximum.vi"("error in"=w1, "camera handle in"=w4) -> ("ExactReadoutCountMaximum"=→"ExactReadoutCountMaximum":i64)  [unwired: 7 in, 2 out]
  n116 = call "Get_ExposureTime.vi"("error in"=w1, "camera handle in"=w4) -> ("ExposureTime (ms)"=→"Exposure Time":dbl)  [unwired: 7 in, 2 out]
  n117 = call "Get_OnlineReadoutRateCalculation.vi"("error in"=w1, "camera handle in"=w4) -> ("OnlineReadoutRateCalculation"=→"OnlineReadoutRateCalculation":dbl)  [unwired: 7 in, 2 out]
  n118 = call "Get_FrameRateCalculation.vi"("error in"=w1, "camera handle in"=w4) -> ("FrameRateCalculation"=→"FrameRateCalculation":dbl)  [unwired: 7 in, 2 out]
  n119 = call "Get_VerticalShiftRate.vi"("error in"=w1, "camera handle in"=w4) -> ("VerticalShiftRate"=→"VerticalShiftRate":dbl)  [unwired: 7 in, 2 out]
  n120 = call "Get_SensorTemperatureSetPoint.vi"("error in"=w1, "camera handle in"=w4) -> ("SensorTemperatureSetPoint"=→"SensorTemperatureSetPoint":dbl)  [unwired: 7 in, 2 out]
  n121 = call "Get_PixelGapHeight.vi"("error in"=w1, "camera handle in"=w4) -> ("PixelGapHeight"=→"PixelGapHeight":dbl)  [unwired: 7 in, 2 out]
  n122 = call "Get_PixelGapWidth.vi"("error in"=w1, "camera handle in"=w4) -> ("PixelGapWidth"=→"PixelGapWidth":dbl)  [unwired: 7 in, 2 out]
  n123 = call "Get_PixelHeight.vi"("error in"=w1, "camera handle in"=w4) -> ("PixelHeight"=→"PixelHeight":dbl)  [unwired: 7 in, 2 out]
  n124 = call "Get_PixelWidth.vi"("error in"=w1, "camera handle in"=w4) -> ("PixelWidth"=→"PixelWidth":dbl)  [unwired: 7 in, 2 out]
  n125 = call "Get_ReadoutRateCalculation.vi"("error in"=w1, "camera handle in"=w4) -> ("ReadoutRateCalculation"=→"ReadoutRateCalculation":dbl)  [unwired: 7 in, 2 out]
  n126 = call "Get_ReadoutTimeCalculation.vi"("error in"=w1, "camera handle in"=w4) -> ("ReadoutTimeCalculation"=→"ReadoutTimeCalculation":dbl)  [unwired: 7 in, 2 out]
  n127 = call "Get_SensorTemperatureReading.vi"("error in"=w1, "camera handle in"=w4) -> ("SensorTemperatureReading"=→"SensorTemperatureReading":dbl)  [unwired: 7 in, 2 out]
  n128 = call "Get_ShutterClosingDelay.vi"("error in"=w1, "camera handle in"=w4) -> ("Shutter Closing Delay"=→"Shutter Closing Delay":dbl)  [unwired: 7 in, 2 out]
  n129 = call "Get_AdcSpeed.vi"("error in"=w1, "camera handle in"=w4) -> ("AdcSpeed"=→"AdcSpeed":dbl)  [unwired: 7 in, 2 out]
  n130 = call "Get_ShutterDelayResolution.vi"("error in"=w1, "camera handle in"=w4) -> ("Shutter Delay Resolution"=→"Shutter Delay Resolution":dbl)  [unwired: 7 in, 2 out]
